vi "majutilisateur.vi"() -> ()   [LabVIEW 2015]
uses:
  <vilib>/httpClient/LabVIEWHTTPClient.lvlib
panel:
  in  "OK Button 4":bool
  in  "OK Button 3":bool
  in  "String 3":string
  in  "String 5":string
  in  "String 4":string
  in  "String 2":string
  in  "String":string
  in  "Combo Box":string(combo)
  in  "OK Button 2":bool
  in  "OK Button":bool
  # "Choisir  Cin utilisateur"
  # "Nom utilisateur"
  # "GSM utilisateur"
  # "Email utilisateur"
  # "Login utilisateur"
  # "Mot de passe utilisateur"
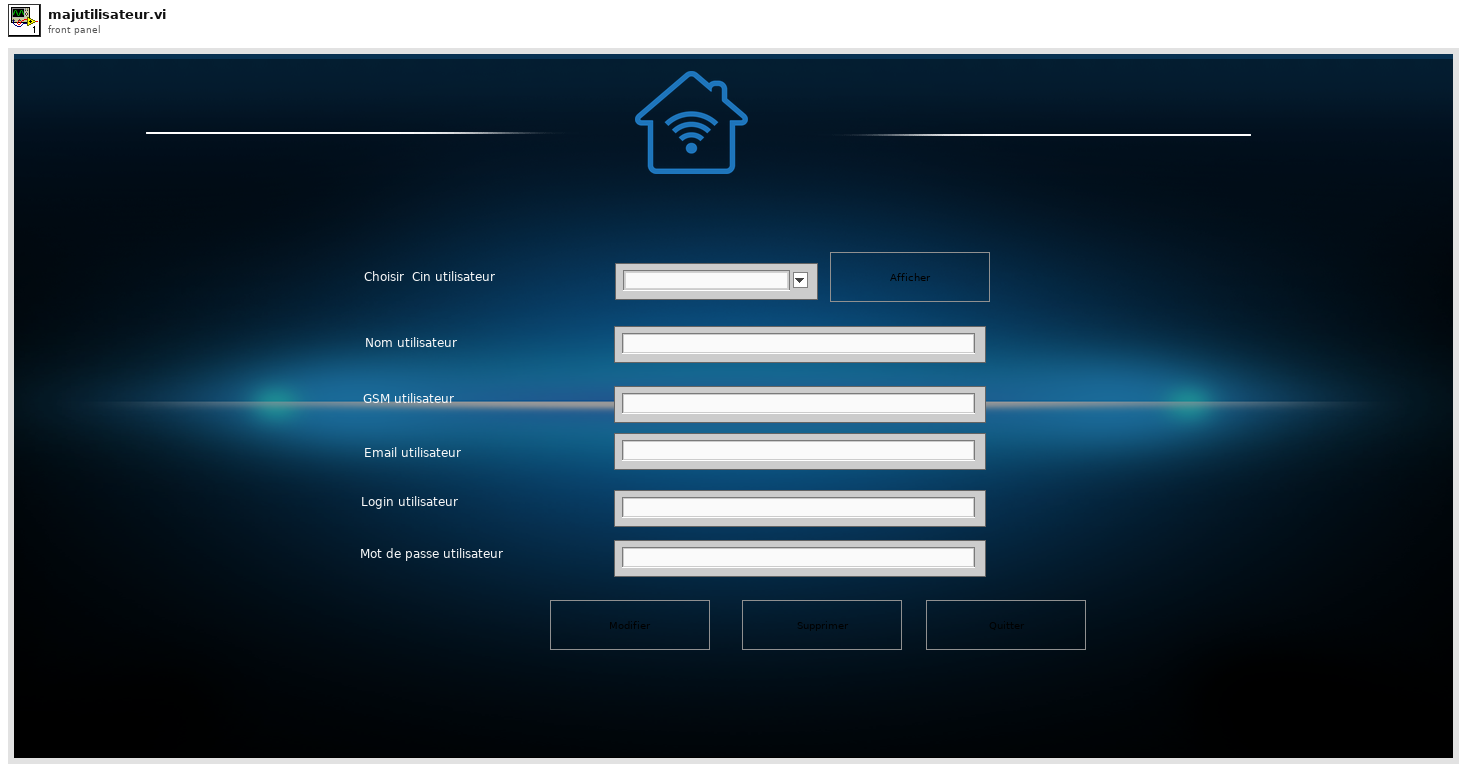
[diagram p1: front panel]
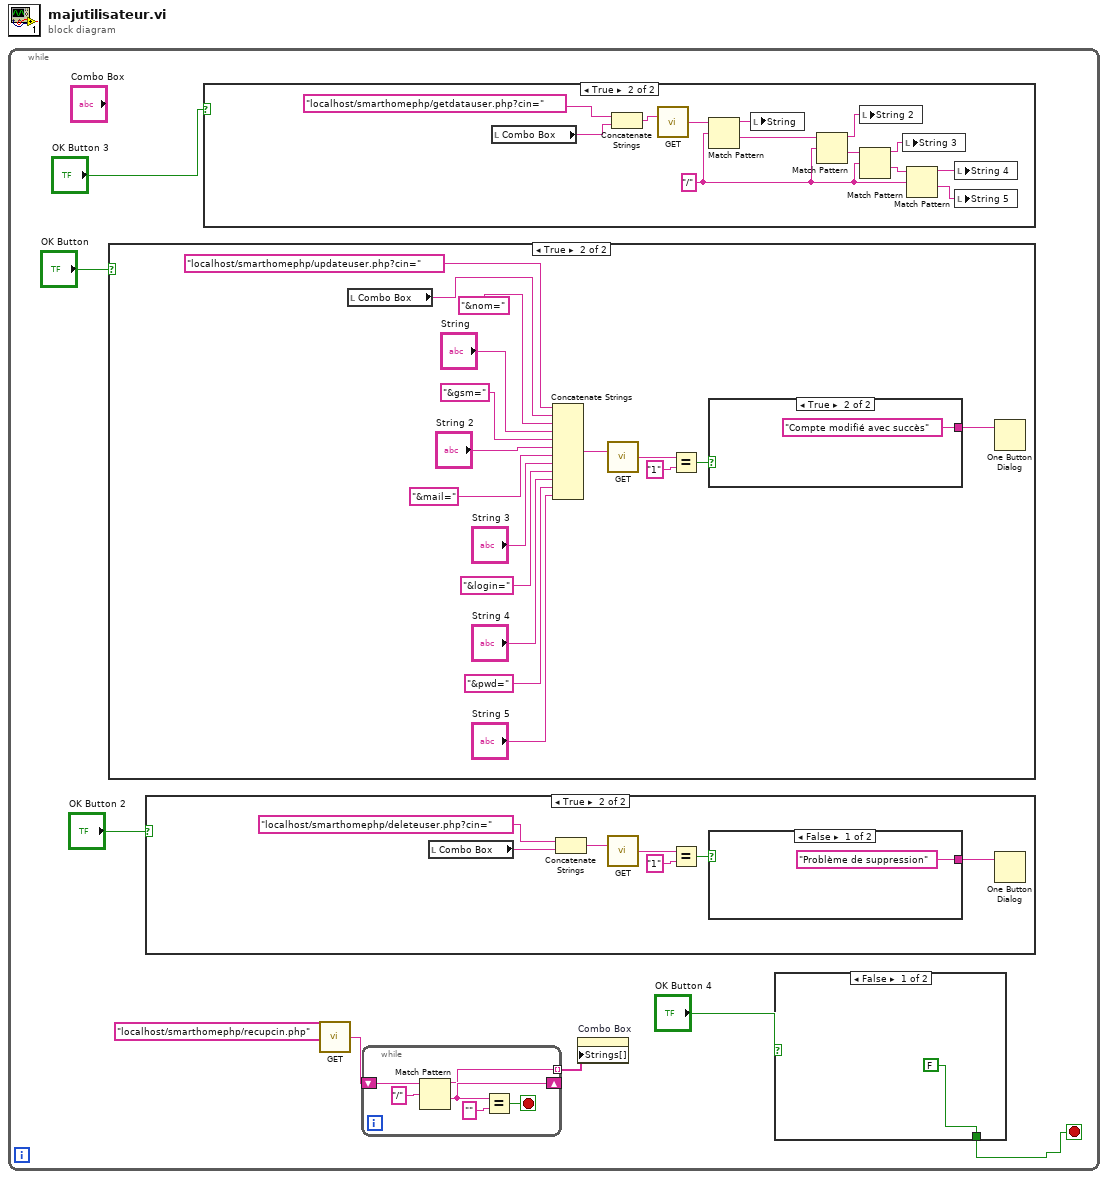
[diagram p0: block diagram]
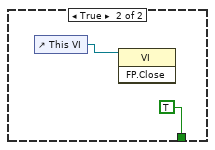
[diagram p2: hidden frame]
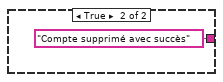
[diagram p4: hidden frame]
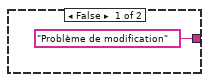
[diagram p6: hidden frame]
diagram:
  n1 = while {
    stop <- w1 stop-if-true
    n2 = case shown="True" "OK Button" {
      frame False {
      }
      frame True {
        n3 = local read "Combo Box"() -> (w42:string)
        n4 = Concatenate Strings("localhost/smarthomephp/updateuser.php?cin=", w42, "&nom=", "String", "&gsm=", "String 2", "&mail=", "String 3", "&login=", "String 4", "&pwd=", "String 5") -> (w31:string)
        n5 = call <vilib>:"GET.vi"("url"=w31) -> ("body"=w30:string)  [unwired: 11 in, 3 out]
        n6 = Equal?(x=w30, y="1") -> (x = y?=w28:bool)
        n7 = case shown="True" w28 {
          tunnel: ["Problème de modification" "Compte modifié avec succès"] -> w27
          frame False {
          }
          frame True {
          }
        }
        n8 = One Button Dialog(message=w27) -> ()  [unwired: 1 in, 1 out]
      }
    }
    n9 = case shown="True" "OK Button 2" {
      frame False {
      }
      frame True {
        n10 = local read "Combo Box"() -> (w19:string)
        n11 = Concatenate Strings("localhost/smarthomephp/deleteuser.php?cin=", w19) -> (w18:string)
        n12 = call <vilib>:"GET.vi"("url"=w18) -> ("body"=w21:string)  [unwired: 11 in, 3 out]
        n13 = Equal?(x=w21, y="1") -> (x = y?=w23:bool)
        n14 = case shown="False" w23 {
          tunnel: ["Problème de suppression" "Compte supprimé avec succès"] -> w24
          frame False {
          }
          frame True {
          }
        }
        n15 = One Button Dialog(message=w24) -> ()  [unwired: 1 in, 1 out]
      }
    }
    n16 = case shown="True" "OK Button 3" {
      frame False {
      }
      frame True {
        w48 = "/" ("regular expression")
        n17 = local read "Combo Box"() -> (w57:string)
        n18 = Concatenate Strings("localhost/smarthomephp/getdatauser.php?cin=", w57) -> (w56:string)
        n19 = call <vilib>:"GET.vi"("url"=w56) -> ("body"=w55:string)  [unwired: 11 in, 3 out]
        n20 = Match Pattern(string=w55, regular expression=w48) -> (before substring=w54:string, after substring=w53:string)  [unwired: 1 in, 2 out]
        n21 = local write "String"(w54) -> ()
        n22 = Match Pattern(string=w53, regular expression=w48) -> (before substring=w52:string, after substring=w51:string)  [unwired: 1 in, 2 out]
        n23 = local write "String 2"(w52) -> ()
        n24 = Match Pattern(string=w51, regular expression=w48) -> (before substring=w50:string, after substring=w49:string)  [unwired: 1 in, 2 out]
        n25 = local write "String 3"(w50) -> ()
        n26 = Match Pattern(string=w49, regular expression=w48) -> (before substring=w47:string, after substring=w46:string)  [unwired: 1 in, 2 out]
        n27 = local write "String 4"(w47) -> ()
        n28 = local write "String 5"(w46) -> ()
      }
    }
    n29 = call <vilib>:"GET.vi"("url"="localhost/smarthomephp/recupcin.php") -> ("body"=w4:string)  [unwired: 11 in, 3 out]
    n30 = while {
      shift-right: [w14] -> _
      shift-left: w4 -> [w16]
      tunnel: [w12] -> w5 mode=indexing
      stop <- w13 stop-if-true
      n31 = Match Pattern(string=w16, regular expression="/") -> (before substring=w12:string, after substring=w14:string)  [unwired: 1 in, 2 out]
      n32 = Equal?(x=w14, y="") -> (x = y?=w13:bool)
    }
    n33 = property on="Combo Box" class="CmbBox"("Strings[]"=w5) -> ()  [unwired: 2 in, 2 out]
    n34 = case shown="False" "OK Button 4" {
      tunnel: [FALSE TRUE] -> w1
      frame False {
      }
      frame True {
        n35 = control-ref of="This VI"() -> (w11:refnum<vi>)
        n36 = invoke class="VI" method="FP.Close"(reference=w11) -> ()  [unwired: 2 in, 3 out]
      }
    }
  }
